vi "BuildMoveCommand.vi"(1 "Relative/Absolute\nPosition":enum16{"Relative", "Absolute"}(ring), 2 "Position Counts":i32, 3 "Speed Counts":i32, 4 "Axis":enum16{"Z", "Y", "X"}(ring)) -> (0 "Command Strings":string[](array[string]))   [LabVIEW 2023]
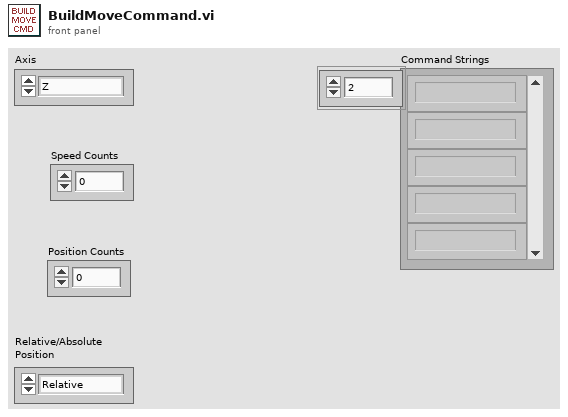
[diagram p1: front panel]
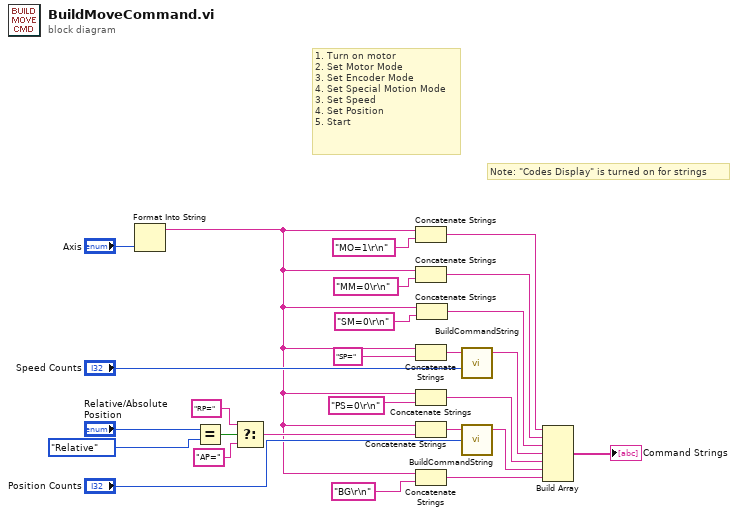
[diagram p0: block diagram]
diagram:
  # "Note: \"Codes Display\" is turned on for strings"
  # "1. Turn on motor\n2. Set Motor Mode\n3. Set Encoder Mode\n4. Set Special Motion Mode\n3. Set Speed\n4. Set Position\n5. Start"
  n1 = Format Into String("Axis") -> (resulting string=w3:string)  [unwired: 3 in, 1 out]
  n2 = Equal?(x="Relative/Absolute\nPosition", y=enum16{"Relative", "Absolute"}."Relative" ("Relative/Absolute\nPosition")) -> (x = y?=w21:bool)
  n3 = Select(t="RP=", s=w21, f="AP=") -> (s? t:f=w16:string)
  n4 = Concatenate Strings(w3, "MO=1\r\n") -> (w5:string)
  n5 = Concatenate Strings(w3, "MM=0\r\n") -> (w2:string)
  n6 = Concatenate Strings(w3, "SP=") -> (w23:string)
  n7 = Concatenate Strings(w3, "PS=0\r\n") -> (w6:string)
  n8 = Concatenate Strings(w3, w16) -> (w24:string)
  n9 = Concatenate Strings(w3, "BG\r\n") -> (w8:string)
  n10 = Concatenate Strings(w3, "SM=0\r\n") -> (w1:string)
  n11 = call "BuildCommandString.vi"("Numeric Value"="Speed Counts", "Command"=w23) -> ("Result"=w11:string)  [unwired: 2 in, 1 out]
  n12 = call "BuildCommandString.vi"("Numeric Value"="Position Counts", "Command"=w24) -> ("Result"=w7:string)  [unwired: 2 in, 1 out]
  n13 = Build Array(w5, w2, w1, w11, w6, w7, w8) -> (→"Command Strings":string[])
